vi "Generic command handler.vi"(8 "error in (no error)":errorcluster, 10 "Message in":refnum<class "GenericMessage.lvclass">, 11 "Cobolt in":refnum<class "Cobolt.lvclass">) -> (0 "error out":errorcluster, 2 "command":string, 3 "Cobolt out":refnum<class "Cobolt.lvclass">)   [LabVIEW 2012, in "Cobolt.lvclass"]
doc: "The generic_command_handler processes the command 'generic'. Commands which are not part of the predefined list of commands fall under the 'generic' command for special activity."
uses:
  Cobolt.lvclass
  <vilib>/Distrio/Murmex/GenericMessage/GenericMessage.lvclass
  <vilib>/Distrio/Murmex/Murmex/Murmex.lvclass
  Cobolt.lvclass/Cobolt.ctl
  CoboltLaserDrivers_Public_LV2012/CoboltLaser_Controls/ExpectedResponseType.ctl
panel:
  # "This method is called when the GENERIC\ntrigger is sent. \n\nOverride this method when your component needs to\nrespond to this trigger. \n\nCall parent for proper implementation"
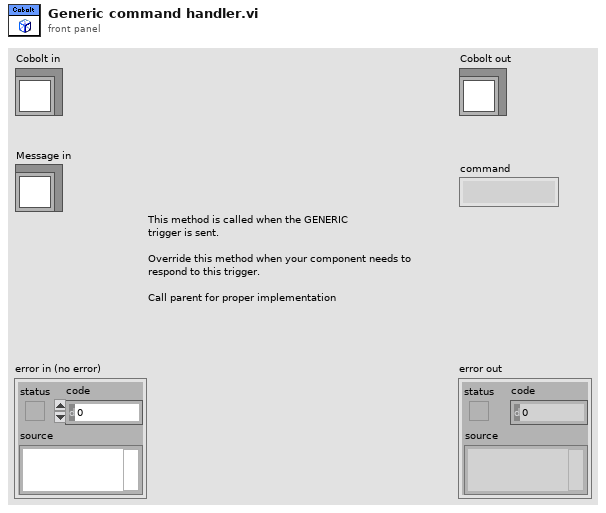
[diagram p1: front panel]
types:
  T1 = typedef "Cobolt.lvclass/ExpectedResponseType.ctl" = u16
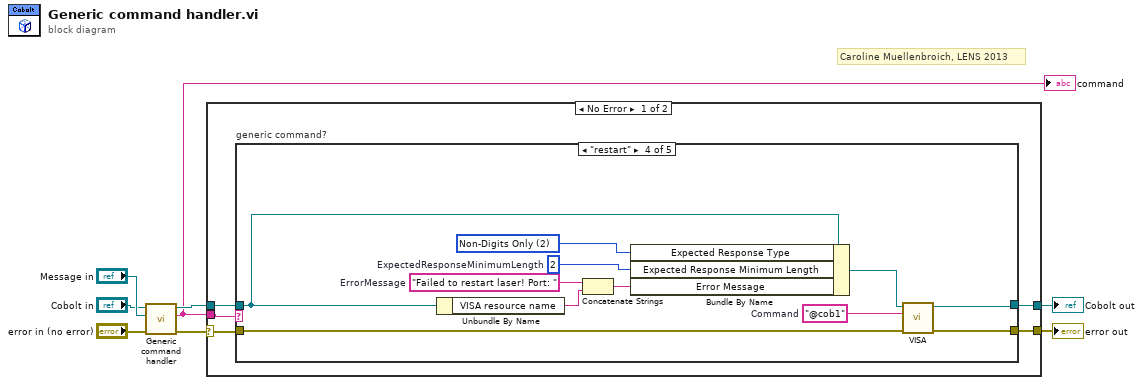
[diagram p0: block diagram]
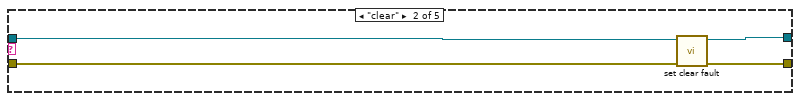
[diagram p3: hidden frame]
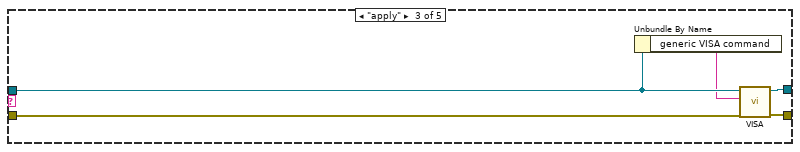
[diagram p4: hidden frame]
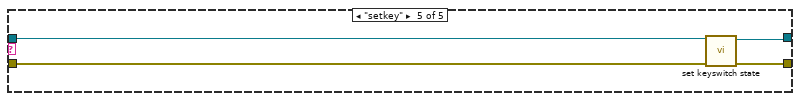
[diagram p5: hidden frame]
diagram:
  # "Caroline Muellenbroich, LENS 2013"
  n1 = call-parent "Generic command handler.vi"("error in (no error)"="error in (no error)", "Message in"="Message in", "Murmex in"="Cobolt in") -> ("error out"=w5:errorcluster, "value"=w2:string, "Murmex out"=w3:refnum<class "Cobolt.lvclass">)  [unwired: 6 in]
  "command" <- w2
  n2 = case shown="No Error" w5 {
    selector: w5 -> [w13 w41]
    tunnel: [w12 w41] -> w4
    tunnel: w3 -> [w10 w40]
    tunnel: [w9 w40] -> w1
    tunnel: w2 -> [w11 _]
    frame No Error {
      n3 = case "generic command?" shown="\"restart\"" w11 {
        tunnel: [w15 w18 w20 w26 w38] -> w12
        tunnel: w13 -> [w15 w19 w21 w30 w39]
        tunnel: [w14 w17 w22 w25 w36] -> w9
        tunnel: w10 -> [w14 w16 w24 w29 w37]
        frame Default {
        }
        frame "clear" {
          n4 = call-dynamic "set clear fault.vi"("error in (no error)"=w19, "Cobolt in"=w16) -> ("error out"=w18:errorcluster, "Cobolt out"=w17:refnum<class "Cobolt.lvclass">)  [unwired: 8 in]
        }
        frame "apply" {
          n5 = Unbundle By Name(w24) -> ("generic VISA command"=w23:string)
          n6 = call-dynamic "VISA.vi"("error in (no error)"=w21, "string to write"=w23, "Cobolt in"=w24) -> ("error out"=w20:errorcluster, "Cobolt out"=w22:refnum<class "Cobolt.lvclass">)  [unwired: 6 in, 1 out]
        }
        frame "restart" {
          w27 = "@cob1"  # Command
          w32 = T1 2 items=["Any", "Digits Only", "Non-Digits Only"] ("ExpectedResponseType")
          w33 = 2  # ExpectedResponseMinimumLength
          w35 = "Failed to restart laser! Port: "  # ErrorMessage
          n7 = Unbundle By Name(w29) -> ("VISA resource name"=w31:string)
          n8 = Concatenate Strings(w35, w31) -> (w34:string)
          n9 = Bundle By Name(cluster=w29, "Expected Response Type"=w32, "Expected Response Minimum Length"=w33, "Error Message"=w34) -> (w28:refnum<class "Cobolt.lvclass">)
          n10 = call-dynamic "VISA.vi"("error in (no error)"=w30, "string to write"=w27, "Cobolt in"=w28) -> ("error out"=w26:errorcluster, "Cobolt out"=w25:refnum<class "Cobolt.lvclass">)  [unwired: 6 in, 1 out]
        }
        frame "setkey" {
          n11 = call-dynamic "set keyswitch state.vi"("error in (no error)"=w39, "Cobolt in"=w37) -> ("error out"=w38:errorcluster, "Cobolt out"=w36:refnum<class "Cobolt.lvclass">)  [unwired: 8 in]
        }
      }
    }
    frame Error {
    }
  }
  "error out" <- w4
  "Cobolt out" <- w1
